vi "YKMW100 VF0 Relay Status.vi"(0 "MW100":refnum<visa-resource-name>, 11 "Error In":errorcluster) -> (4 "MW100 Out":refnum<visa-resource-name>, 6 "Module 4 Relay Status":T1, 8 "DO Card Detected for Module 5":bool, 10 "Read Array":string[](array[string]), 15 "error out":errorcluster)   [LabVIEW 2019]
doc: "This VI sends the message. Then it returns the response."
uses:
  Type Definitions/HEWH Module 4 Relay Status.ctl
panel:
  # "POWER:TRUE = OFF"
  # "FALSE = CONTACT CLOSED"
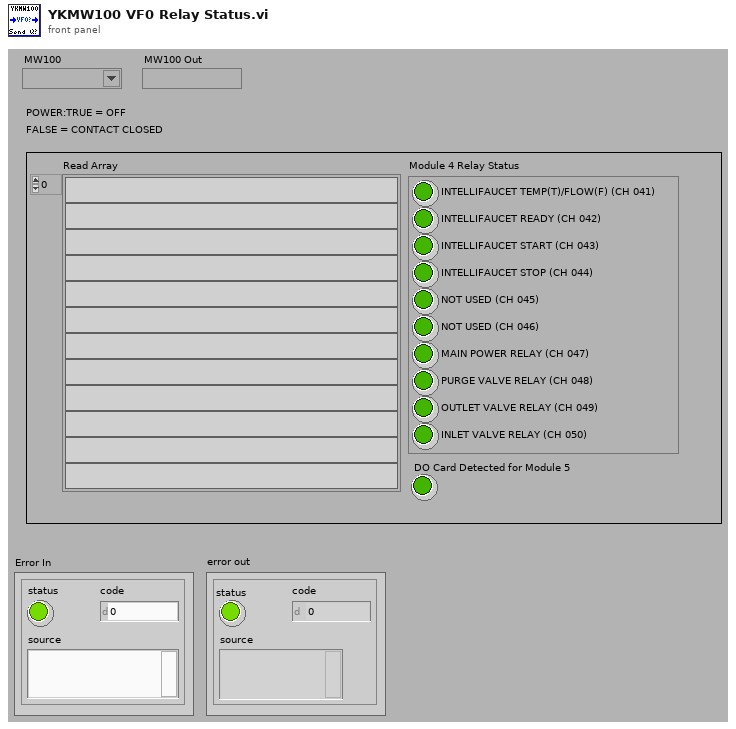
[diagram p1: front panel]
types:
  T1 = typedef "HEWH Module 4 Relay Status.ctl" = cluster{"INTELLIFAUCET TEMP(T)/FLOW(F) (CH 041)":bool, "INTELLIFAUCET READY (CH 042)":bool, "INTELLIFAUCET START (CH 043)":bool, "INTELLIFAUCET STOP (CH 044)":bool, "MAIN POWER RELAY (CH 047)":bool, "NOT USED (CH 045)":bool, "NOT USED (CH 046)":bool, "PURGE VALVE RELAY (CH 048)":bool, "OUTLET VALVE RELAY (CH 049)":bool, "INLET VALVE RELAY (CH 050)":bool}
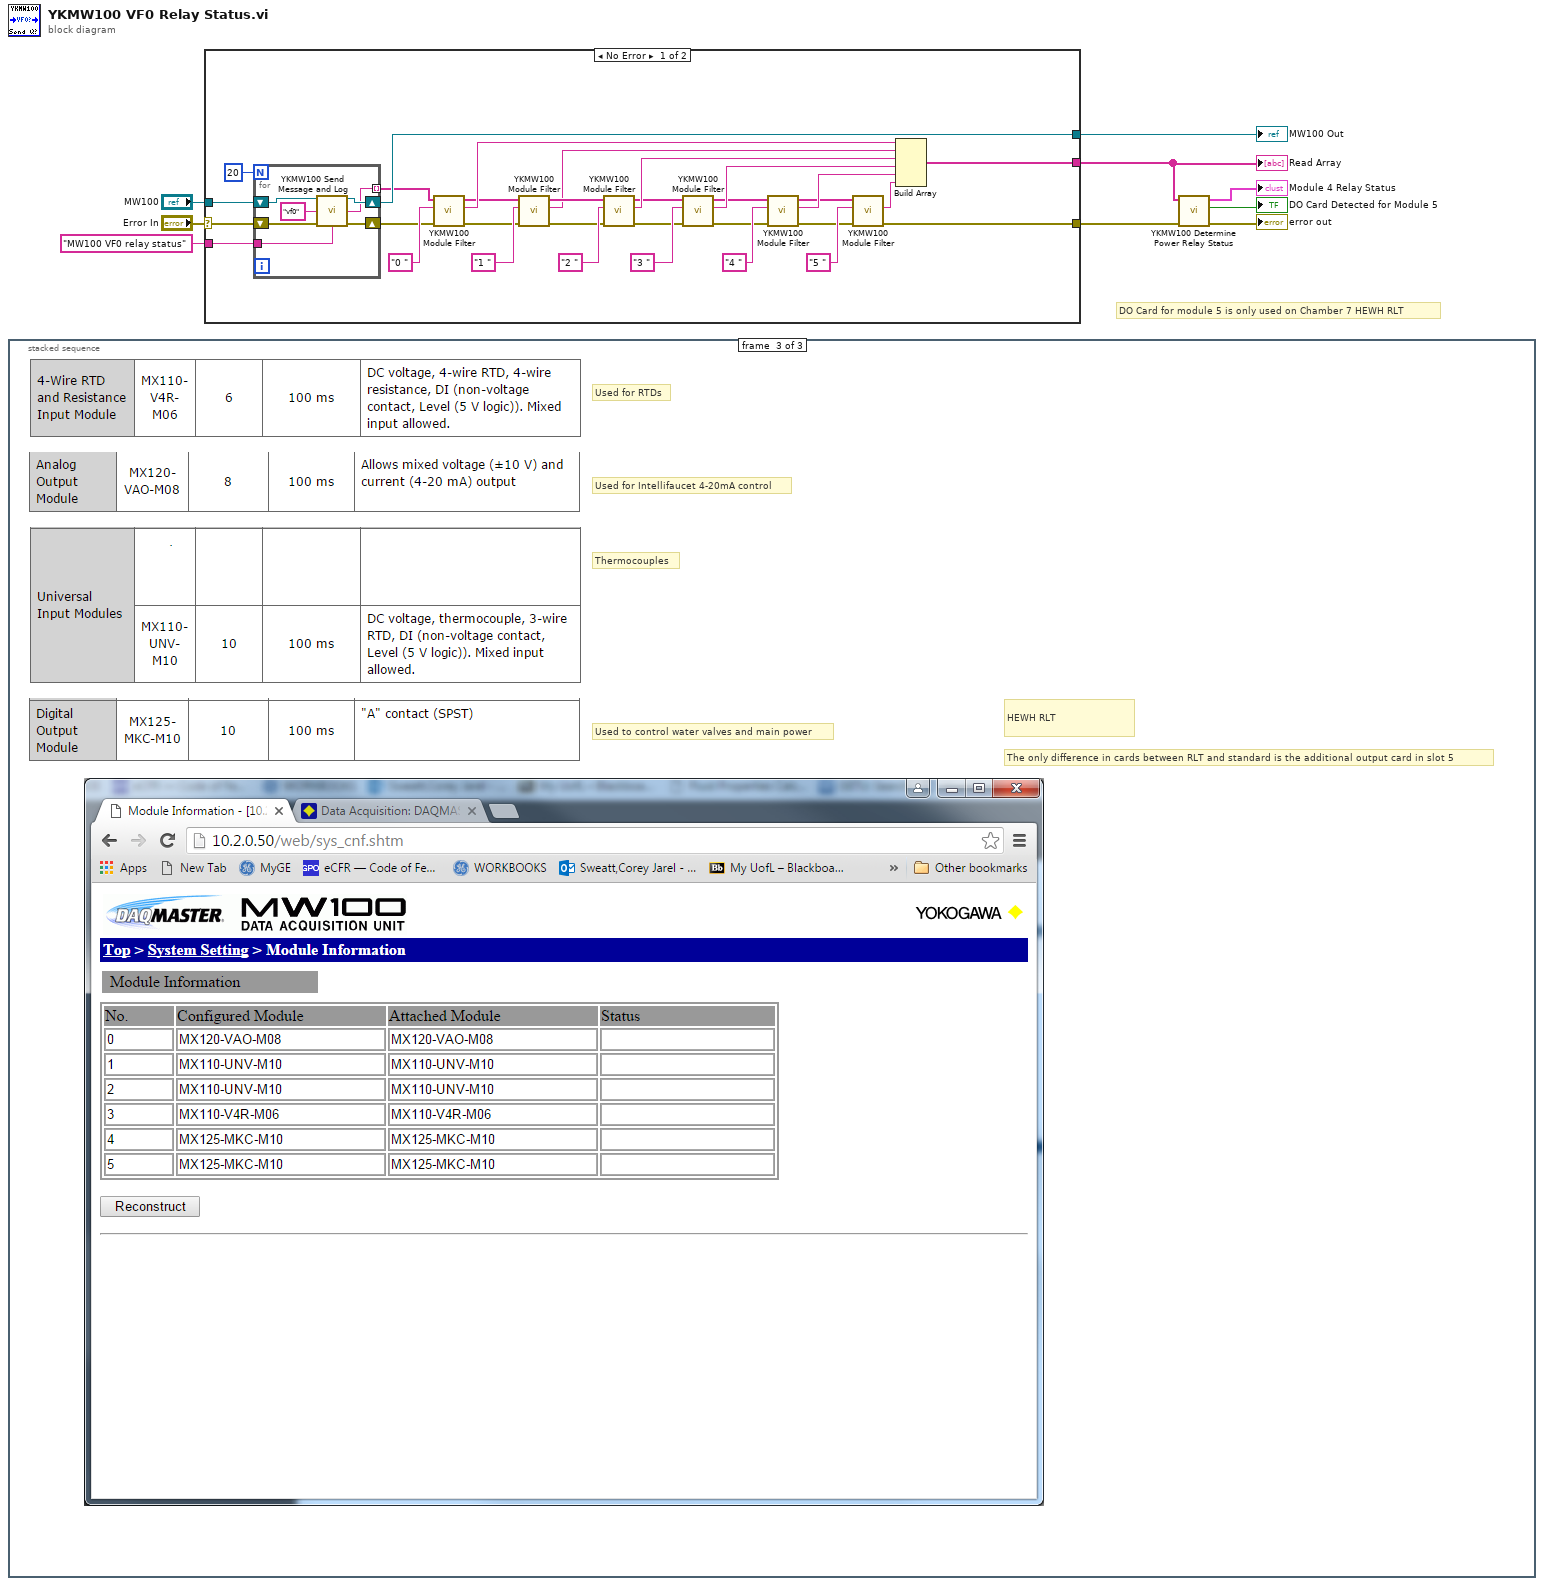
[diagram p0: block diagram]
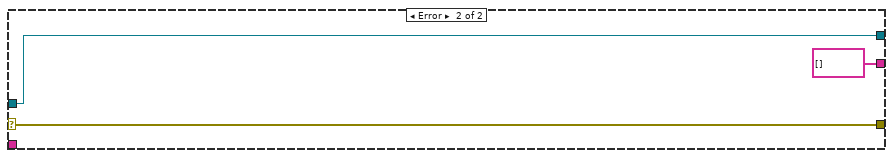
[diagram p4: hidden frame]
diagram:
  # "DO Card for module 5 is only used on Chamber 7 HEWH RLT"
  n1 = stacked-sequence {
    frame #0 {
    }
    frame #1 {
      # "Used to control water valves and main power"
      # "Used for RTDs"
      # "Thermocouples"
      # "Used for Intellifaucet 4-20mA control"
      # "HEWH (Standard)"
    }
    frame #2 {
      # "The only difference in cards between RLT and standard is the additional output card in slot 5"
      # "Used to control water valves and main power"
      # "Used for RTDs"
      # "Thermocouples"
      # "Used for Intellifaucet 4-20mA control"
      # "HEWH RLT"
    }
  }
  n2 = case "no operation if error" shown="No Error" "Error In" {
    selector: "Error In" -> [w36 w48]
    tunnel: "MW100" -> [w37 w50]
    tunnel: [w40 w50] -> w2
    tunnel: [w12 w48] -> w7
    tunnel: [w10 string[] []] -> w3
    tunnel: "MW100 VF0 relay status" ("Source (\"\")") -> [w38 _]
    frame No Error {
      n3 = for {
        N: 20 ("Numeric 4") -> [_]
        tunnel: w38 -> [w47]
        shift-right: [w43] -> w40
        shift-left: w37 -> [w45]
        shift-right: [w41] -> w13
        shift-left: w36 -> [w44]
        tunnel: [w42] -> w14 mode=indexing
        n4 = call "YKMW100 Send Message and Log.vi"("VISA session"=w45, "Send Message (\"\")"="vf0" ("Send Message (\"\")"), "error in (no error)"=w44, "Source (\"\")"=w47) -> ("dup VISA session"=w43:refnum<visa-resource-name>, "Read Buffer"=w42:string, "error out"=w41:errorcluster)  [unwired: 9 in]
      }
      n5 = call "YKMW100 Module Filter.vi"("Error In"=w13, "Select Module"="0 ", "All Data Input"=w14) -> ("Error Out"=w16:errorcluster, "Specific Point"=w31:string, "All Data Output"=w21:string[])  [unwired: 6 in]
      n6 = call "YKMW100 Module Filter.vi"("Error In"=w16, "Select Module"="1 " ("Read Buffer"), "All Data Input"=w21) -> ("Error Out"=w17:errorcluster, "Specific Point"=w11:string, "All Data Output"=w22:string[])  [unwired: 6 in]
      n7 = call "YKMW100 Module Filter.vi"("Error In"=w17, "Select Module"="2 " ("Read Buffer"), "All Data Input"=w22) -> ("Error Out"=w18:errorcluster, "Specific Point"=w32:string, "All Data Output"=w23:string[])  [unwired: 6 in]
      n8 = call "YKMW100 Module Filter.vi"("Error In"=w18, "Select Module"="3 " ("Read Buffer"), "All Data Input"=w23) -> ("Error Out"=w19:errorcluster, "Specific Point"=w33:string, "All Data Output"=w24:string[])  [unwired: 6 in]
      n9 = call "YKMW100 Module Filter.vi"("Error In"=w19, "Select Module"="4 " ("Read Buffer"), "All Data Input"=w24) -> ("Error Out"=w20:errorcluster, "Specific Point"=w34:string, "All Data Output"=w25:string[])  [unwired: 6 in]
      n10 = call "YKMW100 Module Filter.vi"("Error In"=w20, "Select Module"="5 " ("Read Buffer"), "All Data Input"=w25) -> ("Error Out"=w12:errorcluster, "Specific Point"=w35:string)  [unwired: 6 in, 1 out]
      n11 = Build Array(w31, w11, w32, w33, w34, w35) -> (w10:string[])
    }
    frame Error {
    }
  }
  "Read Array" <- w3
  "MW100 Out" <- w2
  n12 = call "YKMW100 Determine Power Relay Status.vi"("Error In"=w7, "Full Module List"=w3) -> ("Error Out"=→"error out":errorcluster, "DO Card Detected for Module 5"=→"DO Card Detected for Module 5":bool, "Module 4 Relay Status"=→"Module 4 Relay Status":T1)  [unwired: 7 in]
